vi "InitializeWaypoint.vi"(1 "Done?":bool, 2 "Tolerance (meters?)":dbl, 3 "Coords":T1 {"North" format="%#_10f"; "East" format="%#_8f"}) -> (0 "Waypoint Out":refnum<class "Waypoint.lvclass">)   [LabVIEW 2012, in "Waypoint.lvclass"]
uses:
  Waypoint.lvclass
  Data/TypeDefs/UTM Location.ctl
  Waypoint.lvclass/Waypoint.ctl
panel:
  out "Error Out":errorcluster
  in  "Error In":errorcluster
  in  "Waypoint In":refnum<class "Waypoint.lvclass">
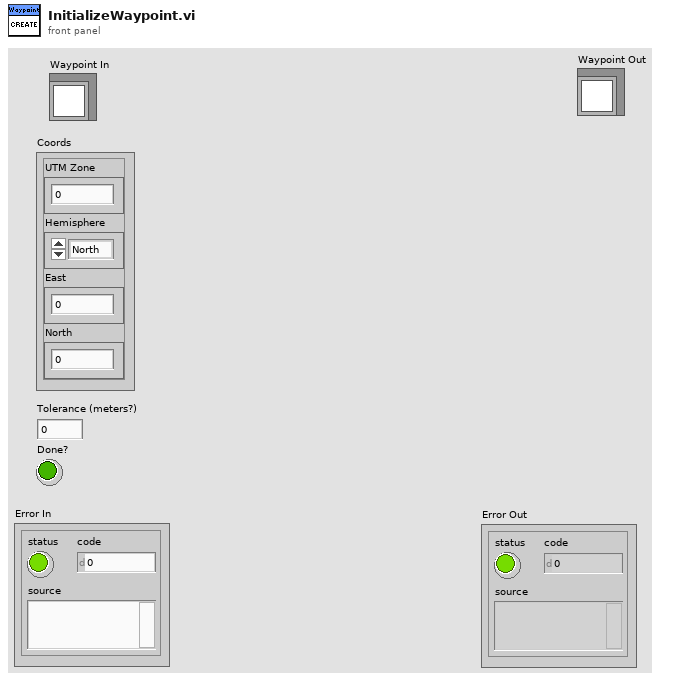
[diagram p1: front panel]
types:
  T1 = typedef "UTM Location.ctl" = cluster{"UTM Zone":dbl, "Hemisphere":enum16{"North", "South"}, "East":dbl, "North":dbl}
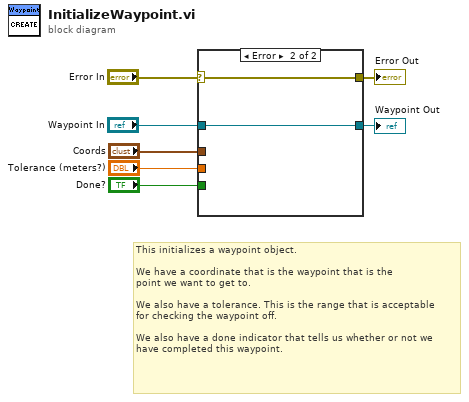
[diagram p0: block diagram]
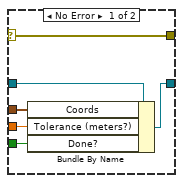
[diagram p2: hidden frame]
diagram:
  # "This initializes a waypoint object. \n\nWe have a coordinate that is the waypoint that is the\npoint we want to get to.\n\nWe also have a tolerance. This is the range that is acceptable\nfor checking the waypoint off. \n\nWe also have a done indicator that tells us whether or not we \nhave completed this waypoint."
  n1 = case shown="Error" "Error In" {
    selector: "Error In" -> [w13 w14]
    tunnel: [w13 w14] -> w6
    tunnel: "Waypoint In" -> [w12 w15]
    tunnel: "Coords" -> [w11 _]
    tunnel: "Tolerance (meters?)" -> [w10 _]
    tunnel: "Done?" -> [w9 _]
    tunnel: [w8 w15] -> w1
    frame No Error {
      n2 = Bundle By Name(cluster=w12, "Coords"=w11, "Tolerance (meters?)"=w10, "Done?"=w9) -> (w8:refnum<class "Waypoint.lvclass">)
    }
    frame Error {
    }
  }
  "Waypoint Out" <- w1
  "Error Out" <- w6
